vi "Table Read & Write.vi"(0 "File Name":string, 1 "Write Table":string[][](table), 2 "File type":string, 3 "error in":errorcluster, 4 "Enum":enum16{"Read", "Write"}(ring), 6 "index":i32=2) -> (8 "Read Table":string[][](array[string]), 10 "error out":errorcluster)   [LabVIEW 2015]
uses:
  Galobal variable_TI.vi
  <vilib>/Utility/file.llb/Read Delimited Spreadsheet (string).vi
  <vilib>/Utility/file.llb/Write Delimited Spreadsheet (string).vi
panel:
  out "element":path
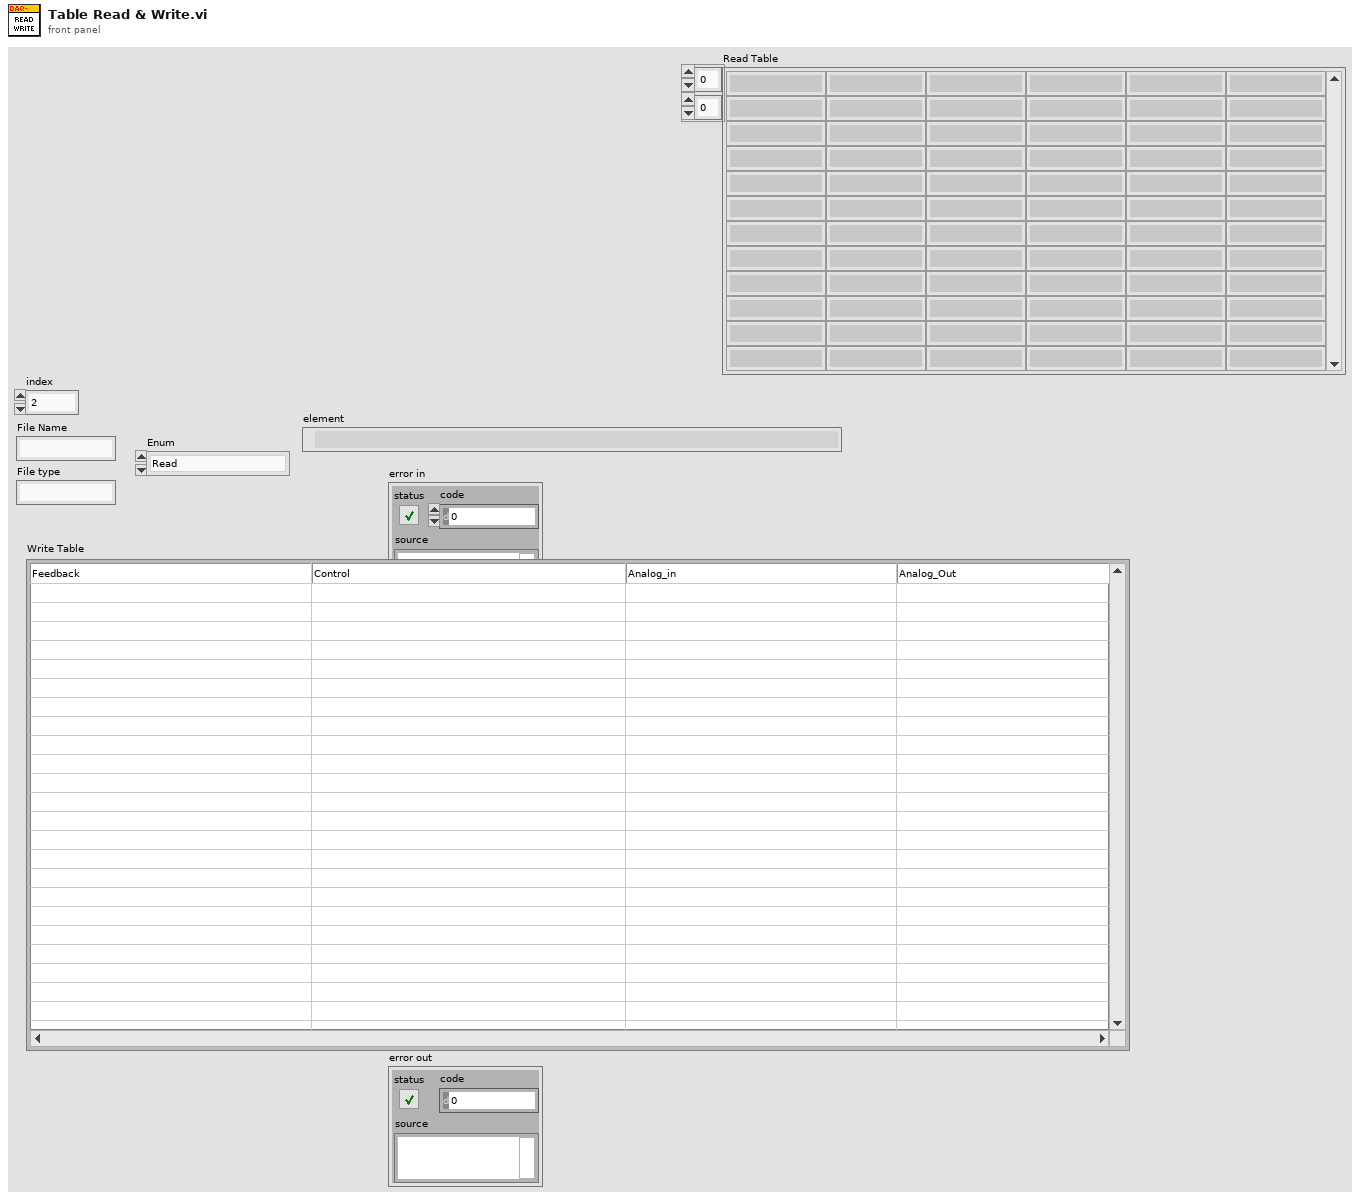
[diagram p1: front panel]
types:
  T1 = enum16{"open", "replace", "create", "open or create", "replace or create", "replace or create with confirmation"}
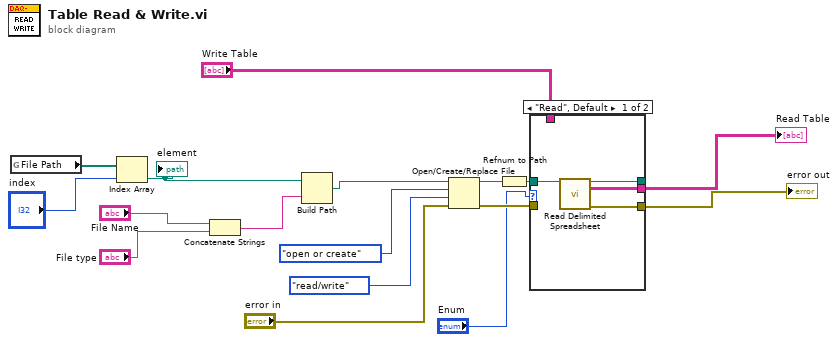
[diagram p0: block diagram]
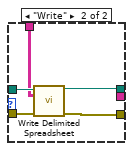
[diagram p2: hidden frame]
diagram:
  n1 = global read "Galobal variable_TI.vi" "File Path"() -> (w17:path[])
  n2 = Index Array(array=w17, index="index") -> (element=w13:path)
  "element" <- w13
  n3 = Concatenate Strings("File Name", "File type") -> (w12:string)
  n4 = Build Path(base path=w13, name or relative path=w12) -> (appended path=w11:path)
  n5 = Open/Create/Replace File(file path (use dialog)=w11, error in="error in", operation (0:open)=T1."open or create", access (0:read/write)=enum16{"read/write", "read-only", "write-only"}."read/write") -> (refnum out=w7:refnum<file>, error out=w5:errorcluster)  [unwired: 2 in, 1 out]
  n6 = Refnum to Path(1:w7) -> (0:w6:path)
  n7 = case shown="\"Read\", Default" "Enum" {
    tunnel: w6 -> [w21 w26]
    tunnel: w5 -> [_ w25]
    tunnel: "Write Table" -> [_ w24]
    tunnel: [w19 w23] -> w2
    tunnel: [w20 w22] -> _
    tunnel: [w18 _] -> w1
    frame "Read", Default {
      n8 = call-poly <vilib>:"Read Delimited Spreadsheet.vi"("file path (dialog if empty)"=w21) -> ("new file path (Not A Path if cancelled)"=w20:path, "all rows"=w18:string[][], "error out"=w19:errorcluster)  [unwired: 9 in, 3 out]
    }
    frame "Write" {
      n9 = call-poly <vilib>:"Write Delimited Spreadsheet.vi"("file path (dialog if empty)"=w26, "2D data"=w24, "error in (no error)"=w25) -> ("new file path (Not A Path if cancelled)"=w22:path, "error out"=w23:errorcluster)  [unwired: 11 in]
    }
  }
  "error out" <- w2
  "Read Table" <- w1
